vi "connect.vi"(8 "error in (no error)":errorcluster, 11 "SMSD in":refnum<class "SMSD.lvclass">) -> (0 "error out":errorcluster, 3 "SMSD out":refnum<class "SMSD.lvclass">)   [LabVIEW 2019, in "SMSD.lvclass"]
uses:
  SMSD.lvclass
  D:/my_projects/projects/Algorithms/Labview/19/Modbus/MB_TCP2/MB_TCP.lvclass
  MB_TCP.lvclass/MB_TCP.ctl
  NI_modbus_upd/TCP/TCP.lvclass/TCP.ctl
  Ctl/ERROR_OR_COMMANT_Type.ctl
  SMSD.lvclass/SMSD.ctl
  <vilib>/Utility/error.llb/Clear Errors.vi
  SMSD_LAN_COMMAND.vi
  NI_modbus_upd/TCP/TCP.lvclass
  MB_TCP.lvclass
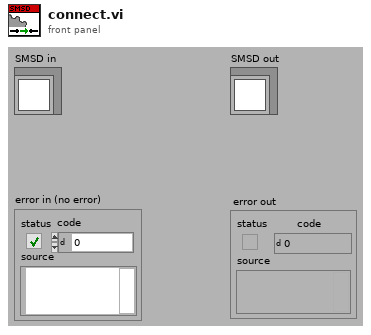
[diagram p1: front panel]
types:
  T1 = typedef "SMSD.lvclass/ERROR_OR_COMMANT_Type.ctl" = enum8{"OK", "OK_ACCESS", "ERROR_ACCESS", "ERROR_ACCESS_TIMEOUT", "ERROR_XOR", "ERROR_NO_COMMAND", "ERROR_LEN", "ERROR_RANGE", "ERROR_WRITE", "ERROR_READ", "ERROR_PROGRAMS", "ERROR_WRITE_SETUP", "NO_NEXT", "END_PROGRAMS", "COMMAND_GET_STATUS_IN_EVENT", "COMMAND_GET_MODE", "COMMAND_GET_ABS_POS", "COMMAND_GET_EL_POS", "COMMAND_GET_SPEED", "COMMAND_GET_MIN_SPEED", "COMMAND_GET_MAX_SPEED", "COMMAND_GET_STACK", "STATUS_RELE_SET", "STATUS_RELE_CLR"}
  T2 = enum8{"CODE_CMD_REQUEST", "CODE_CMD_RESPONSE", "CODE_CMD_POWERSTEP01", "CODE_CMD_POWERSTEP01_W_MEM0", "CODE_CMD_POWERSTEP01_W_MEM1", "CODE_CMD_POWERSTEP01_W_MEM2", "CODE_CMD_POWERSTEP01_W_MEM3", "CODE_CMD_POWERSTEP01_R_MEM0", "CODE_CMD_POWERSTEP01_R_MEM1", "CODE_CMD_POWERSTEP01_R_MEM2", "CODE_CMD_POWERSTEP01_R_MEM3", "CODE_CMD_CONFIG_SET", "CODE_CMD_CONFIG_GET", "CODE_CMD_PASSWORD_SET", "CODE_CMD_ERROR_GET"}
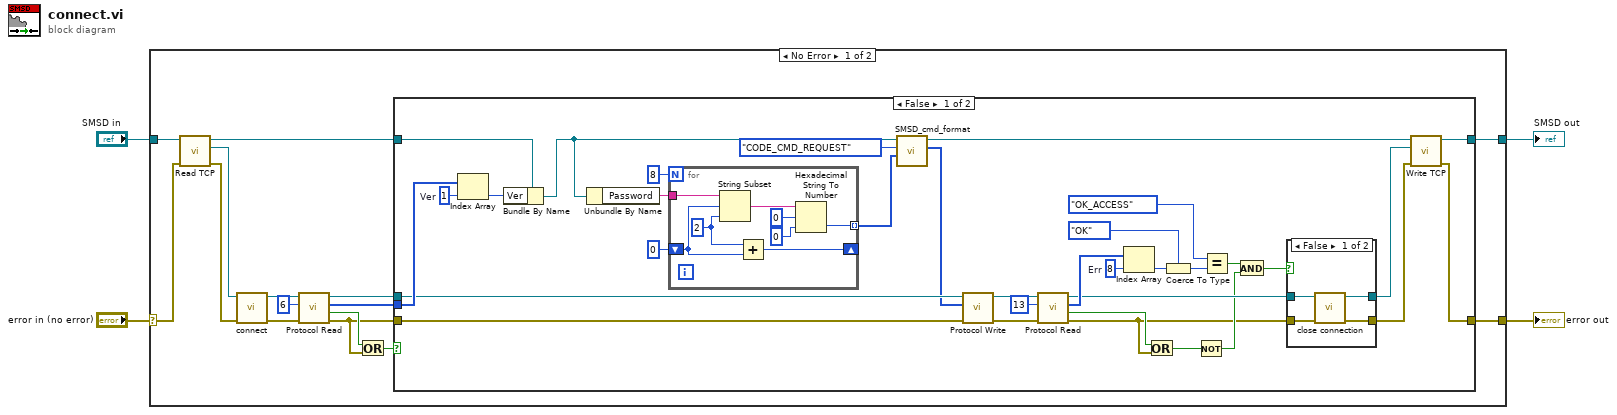
[diagram p0: block diagram]
diagram:
  n1 = case shown="No Error" "error in (no error)" {
    selector: "error in (no error)" -> [w7 w71]
    tunnel: "SMSD in" -> [w10 w70]
    tunnel: [w14 w71] -> w4
    tunnel: [w13 w70] -> w1
    frame No Error {
      n2 = call "Read TCP.vi"("error in (no error)"=w7, "MB_TCP in"=w10) -> ("error out"=w6:errorcluster, "TCP"=w9:refnum<class "TCP.lvclass">, "MB_TCP out"=w8:refnum<class "SMSD.lvclass">)  [unwired: 7 in]
      n3 = call "connect.vi"("error in (no error)"=w6, "TCP in"=w9) -> ("error out"=w17:errorcluster, "TCP out"=w16:refnum<class "TCP.lvclass">)  [unwired: 8 in]
      n4 = call "Protocol Read.vi"("error in (no error)"=w17, "bytes to read"=6, "TCP in"=w16) -> ("error out"=w5:errorcluster, "timed out?"=w12:bool, "data"=w18:u8[], "TCP out"=w15:refnum<class "TCP.lvclass">)  [unwired: 5 in]
      n5 = Or(x=w12, y=w5) -> (x .or. y?=w11:bool)
      n6 = case shown="False" w11 {
        tunnel: w18 -> [w52 _]
        tunnel: w15 -> [w45 _]
        tunnel: w5 -> [w44 w69]
        tunnel: [w21 w69] -> w14
        tunnel: [w23 w68] -> w13
        tunnel: w8 -> [w35 w68]
        frame False {
          w39 = 8  # Err
          w53 = 1  # Ver
          n7 = Index Array(array=w52, index=w53) -> (element=w48:u8)
          n8 = Bundle By Name(cluster=w35, "Ver"=w48) -> (w34:refnum<class "SMSD.lvclass">)
          n9 = Unbundle By Name(w34) -> ("Password"=w49:string)
          n10 = for {
            N: 8 -> [_]
            tunnel: w49 -> [w67]
            tunnel: [w63] -> w46 mode=indexing
            shift-right: [w62] -> _
            shift-left: 0 ("offset (0)") -> [w61]
            w60 = 2 ("y")
            n11 = String Subset(string=w67, offset (0)=w61, length (rest)=w60) -> (substring=w66:string)
            n12 = Add(x=w60, y=w61) -> (x+y=w62:i32)
            n13 = Hexadecimal String To Number(string=w66, offset=0, default (0uL)=u8 0 ("default (0 U32)")) -> (number=w63:u8)  [unwired: 1 out]
          }
          n14 = call "SMSD_cmd_format.vi"("DATA"=w46, "CMD_TYPE"=T2."CODE_CMD_REQUEST", "SMSD in"=w34) -> ("LAN_CMD_out"=w43:u8[], "SMSD out"=w25:refnum<class "SMSD.lvclass">)  [unwired: 7 in]
          n15 = call "Protocol Write.vi"("error in (no error)"=w44, "data"=w43, "protocol layer in"=w45) -> ("error out"=w40:errorcluster, "protocol layer out"=w41:refnum<class "TCP.lvclass">)  [unwired: 6 in, 1 out]
          n16 = call "Protocol Read.vi"("error in (no error)"=w40, "bytes to read"=13, "TCP in"=w41) -> ("error out"=w20:errorcluster, "timed out?"=w30:bool, "data"=w38:u8[], "TCP out"=w31:refnum<class "TCP.lvclass">)  [unwired: 5 in]
          n17 = Index Array(array=w38, index=w39) -> (element=w37:u8)
          n18 = Or(x=w30, y=w20) -> (x .or. y?=w29:bool)
          n19 = Coerce To Type(0:w37, 1:ERROR_OR_COMMANT_Type."OK" ("Ring")) -> (2:w33:T1)
          n20 = Not(x=w29) -> (.not. x?=w27:bool)
          n21 = Equal?(x=ERROR_OR_COMMANT_Type."OK_ACCESS" ("Ring"), y=w33) -> (x = y?=w28:bool)
          n22 = And(x=w28, y=w27) -> (x .and. y?=w26:bool)
          n23 = case shown="False" w26 {
            tunnel: w31 -> [w57 w58]
            tunnel: w20 -> [w56 w59]
            tunnel: [w55 w59] -> w22
            tunnel: [w54 w58] -> w24
            frame False {
              n24 = call "close connection.vi"("error in (no error)"=w56, "TCP in"=w57) -> ("error out"=w55:errorcluster, "TCP out"=w54:refnum<class "TCP.lvclass">)  [unwired: 8 in]
            }
            frame True {
            }
          }
          n25 = call "Write TCP.vi"("error in (no error)"=w22, "TCP"=w24, "MB_TCP in"=w25) -> ("error out"=w21:errorcluster, "MB_TCP out"=w23:refnum<class "SMSD.lvclass">)  [unwired: 7 in]
        }
        frame True {
        }
      }
    }
    frame Error {
    }
  }
  "error out" <- w4
  "SMSD out" <- w1
